vi "Cours2.vi"() -> ()   [LabVIEW 2024]
panel:
  out "Fiche d'ident Read":T1
  in  "Fiche d'ident Write":T1
  in  "new element/subarray":i32
  in  "disabled index (col)":i32
  in  "index (row)":i32
  in  "stop":bool
  out "Resultat":i32[][](array[numeric])
  out "Create Tab":i32[][](array[numeric])
  in  "Array":dbl[][](array[numeric])
  out "x .and. y?":bool[][][][][][][][][](array[boolean])
  in  "TabBool 2":bool[][][][][][][][][](array[boolean])
  in  "TabBool":bool[][][][][][][][][](array[boolean])
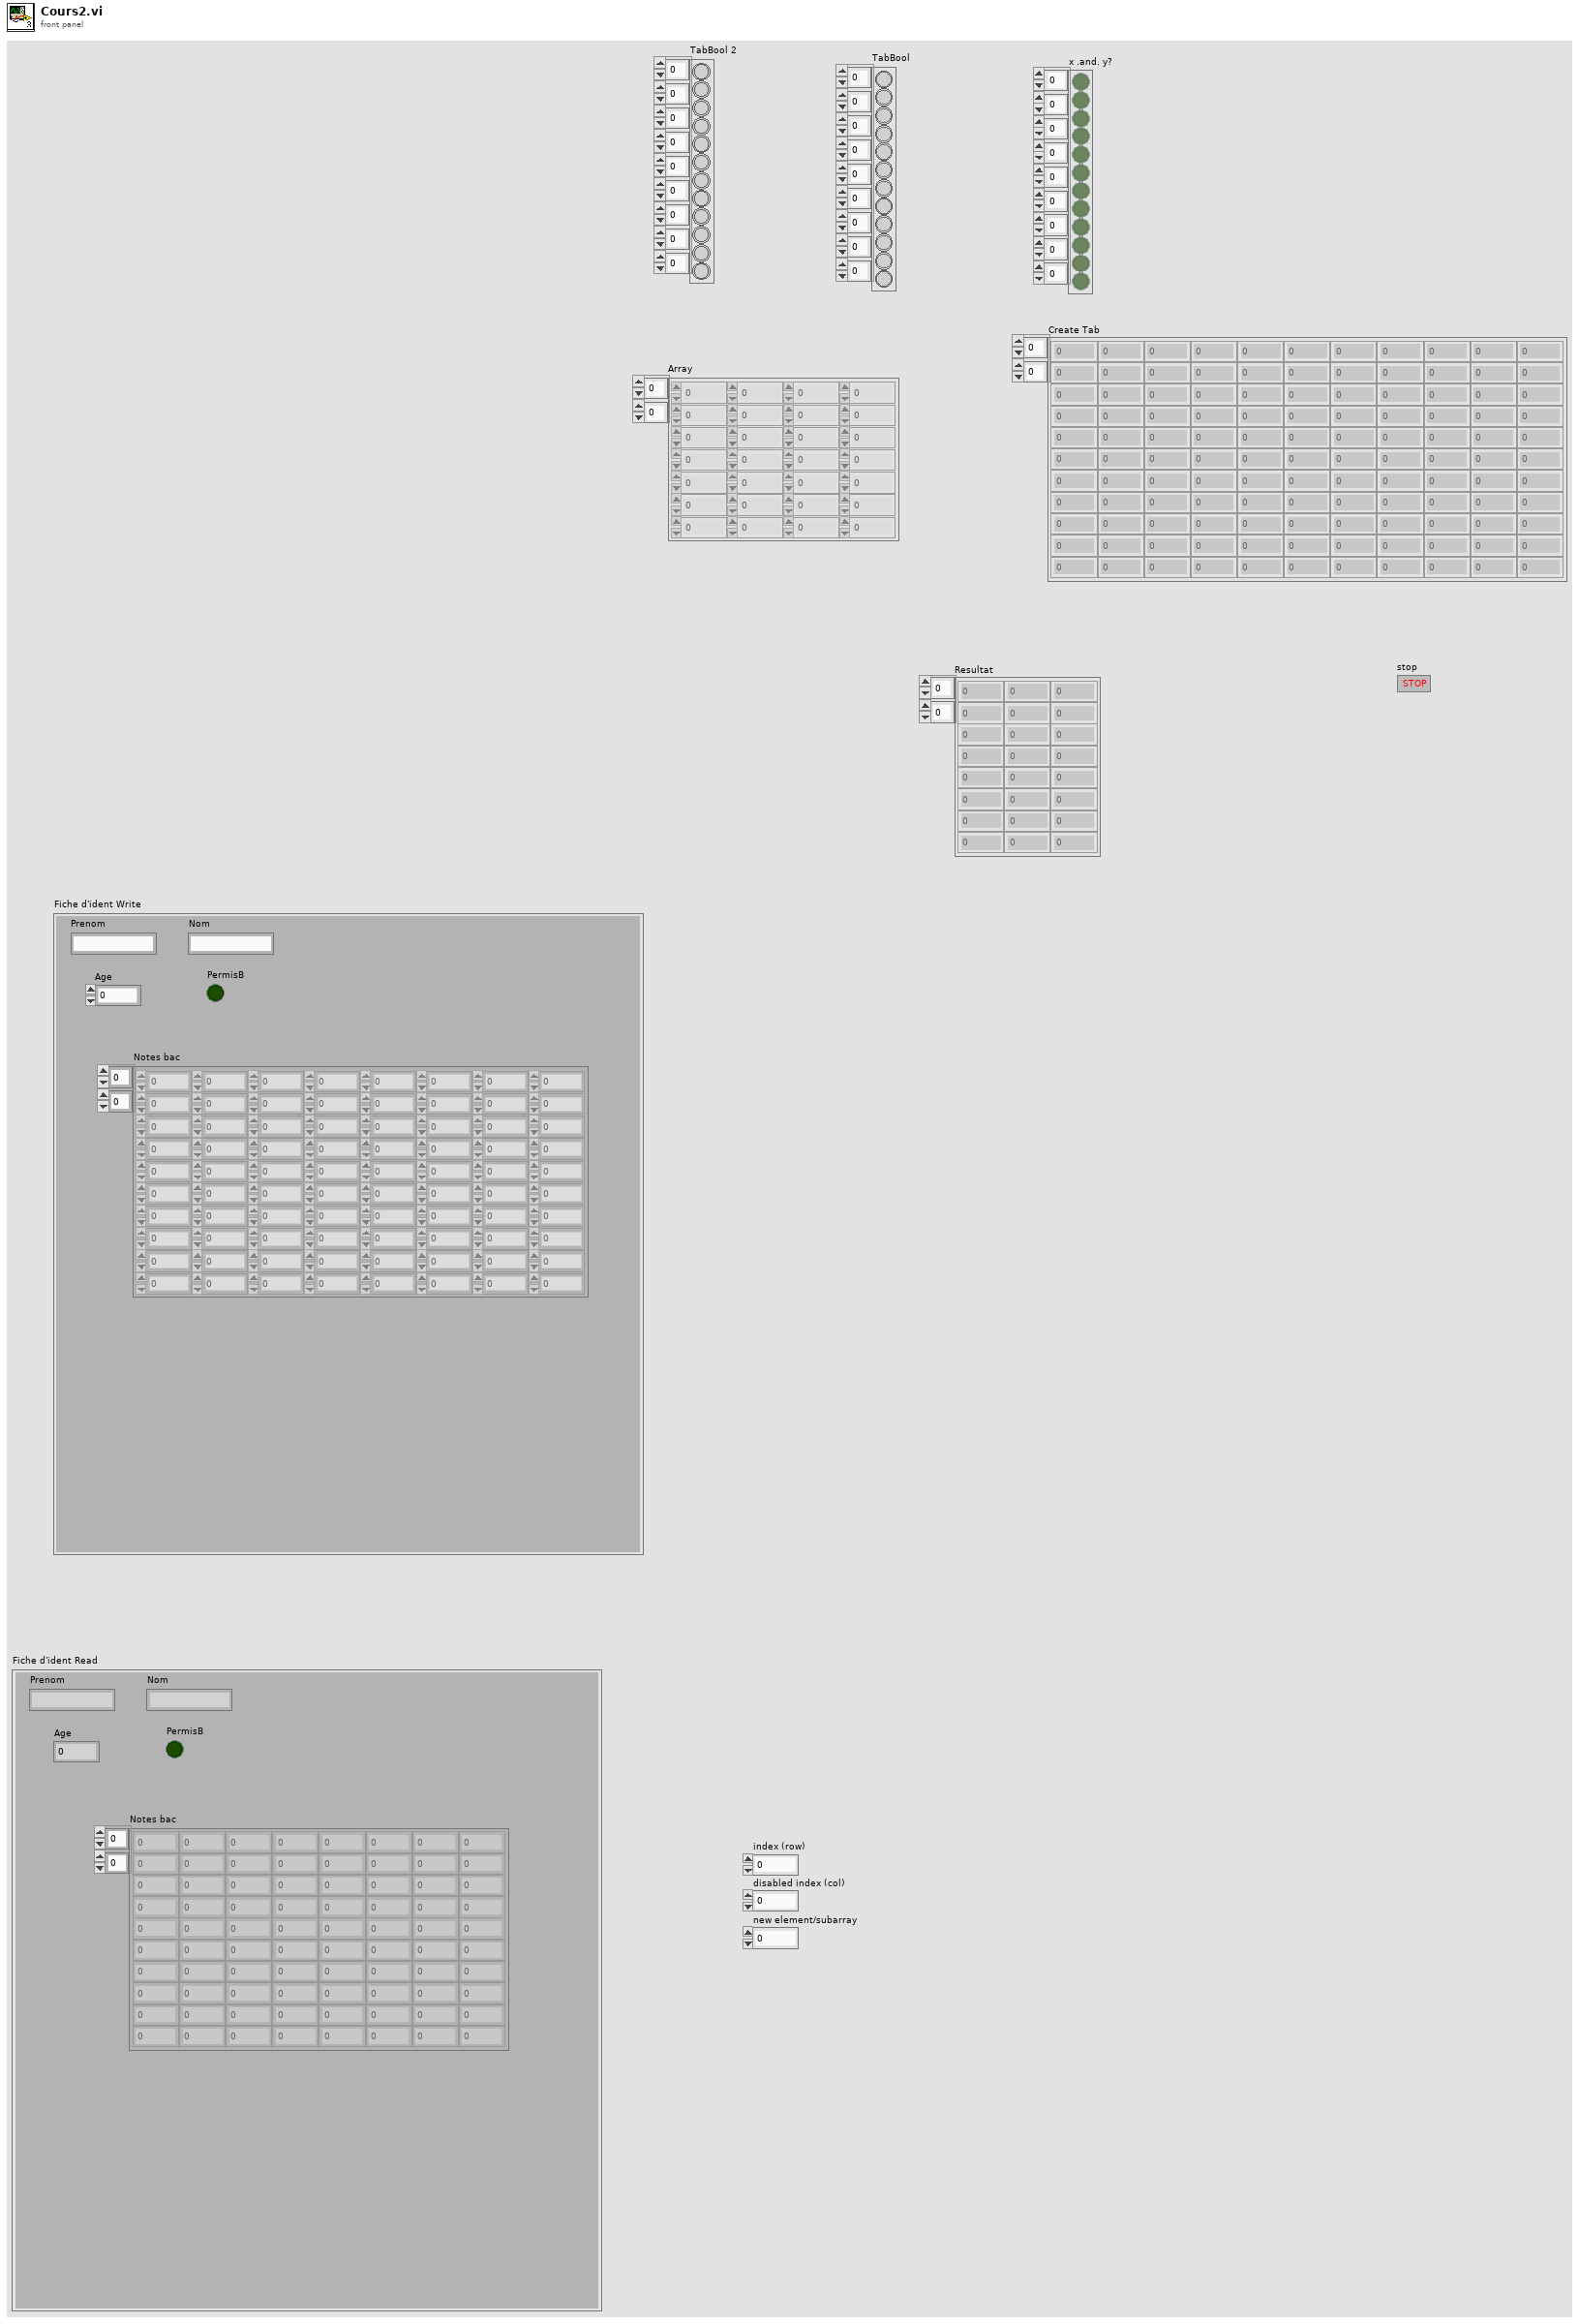
[diagram p1: front panel]
types:
  T1 = cluster{"Prenom":string, "Nom":string, "Age":dbl, "PermisB":bool, "Notes bac":dbl[][]}
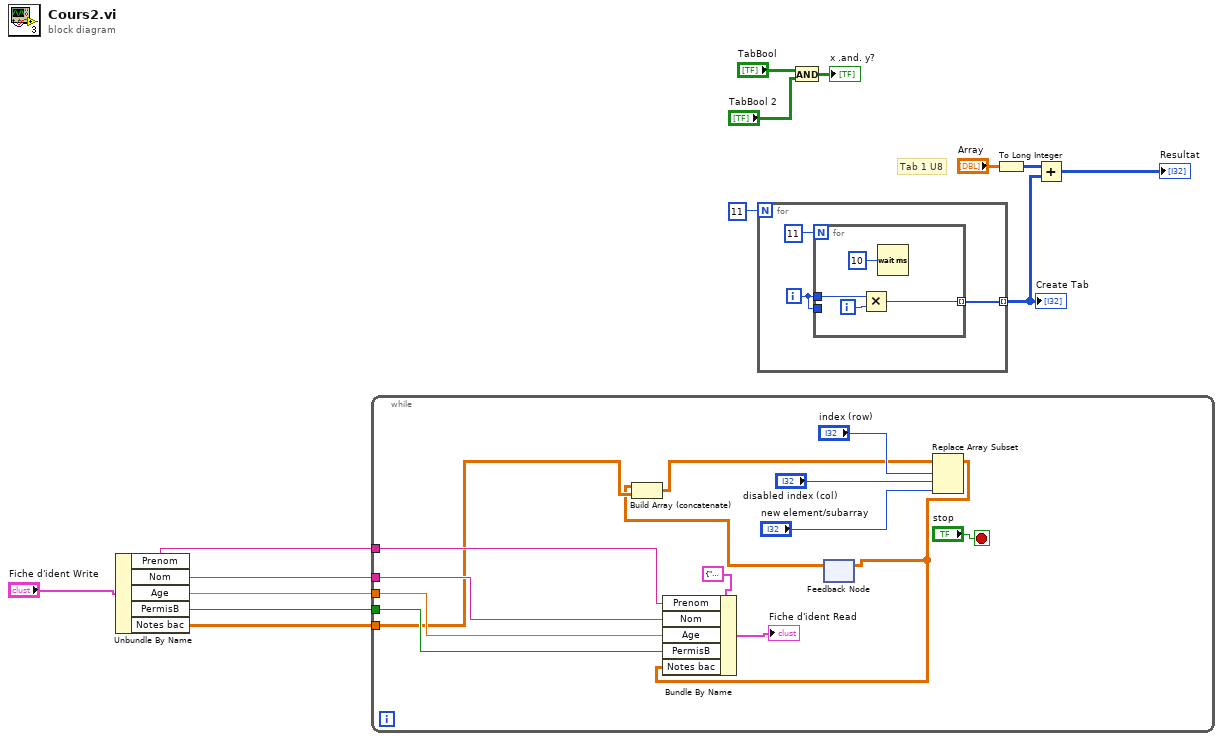
[diagram p0: block diagram]
diagram:
  # "Tab 1 U8"
  n1 = Unbundle By Name("Fiche d'ident Write") -> ("Prenom"=w5:string, "Nom"=w4:string, "Age"=w3:dbl, "PermisB"=w2:bool, "Notes bac"=w1:dbl[][])
  n2 = while {
    tunnel: w5 -> [w22]
    tunnel: w4 -> [w21]
    tunnel: w3 -> [w20]
    tunnel: w2 -> [w19]
    tunnel: w1 -> [w16]
    stop <- "stop" stop-if-true
    n3 = feedback #1() -> (w15:dbl[][])  [unwired: 1 in]
    n4 = Build Array (concatenate)(w15, w16) -> (w18:dbl[][])
    n5 = Replace Array Subset(array=w18, new element="new element/subarray", index (row)="index (row)", index (col)="disabled index (col)") -> (w17:dbl[][])
    n6 = Bundle By Name(cluster=T1 {"Prenom"="0", "Nom"="0", "Age"=0.0, "PermisB"=FALSE, "Notes bac"=[[10.0, 10.0, 10.0, 10.0, 3.0, 10.0, 10.0, 10.0, 10.0, 10.0], [10.0, 10.0, 10.0, 10.0, 3.0, 10.0, 10.0, 10.0, 10.0, 10.0], [10.0, 10.0, 10.0, 10.0, 3.0, 10.0, 10.0, 10.0, 10.0, 10.0], [10.0, 3.0, 3.0, 3.0, 3.0, 3.0, 10.0, 10.0, 10.0, 10.0], [10.0, 10.0, 10.0, 10.0, 3.0, 10.0, 10.0, 10.0, 10.0, 10.0], [10.0, 10.0, 10.0, 10.0, 3.0, 10.0, 10.0, 10.0, 10.0, 10.0], [10.0, 10.0, 10.0, 10.0, 3.0, 10.0, 10.0, 10.0, 10.0, 10.0], [10.0, 10.0, 10.0, 10.0, 10.0, 10.0, 10.0, 10.0, 10.0, 10.0], [10.0, 10.0, 10.0, 10.0, 10.0, 10.0, 10.0, 10.0, 10.0, 10.0], [10.0, 10.0, 10.0, 10.0, 10.0, 10.0, 10.0, 10.0, 10.0, 10.0]]} ("Fiche d'ident Write"), "Prenom"=w22, "Nom"=w21, "Age"=w20, "PermisB"=w19, "Notes bac"=w17) -> (→"Fiche d'ident Read":T1)
    n7 = feedback-in #1(w17) -> ()
  }
  n8 = for {
    N: 11 -> [_]
    tunnel: [w30] -> w10 mode=indexing
    i -> [w29]
    n9 = for {
      N: 11 -> [_]
      tunnel: w29 -> [w35]
      tunnel: [w32] -> w30 mode=indexing
      tunnel: w29 -> [_]
      i -> [w33]
      n10 = Multiply(x=w35, y=w33) -> (x*y=w32:i32)
      n11 = Wait (ms)(milliseconds to wait=u32 10) -> ()  [unwired: 1 out]
    }
  }
  "Create Tab" <- w10
  n12 = And(x="TabBool", y="TabBool 2") -> (x .and. y?=→"x .and. y?":bool[][][][][][][][][])
  n13 = To Long Integer(number="Array") -> (32bit integer=w8:i32[][])
  n14 = Add(x=w8, y=w10) -> (x+y=→"Resultat":i32[][])
